vi "specu1a 1.0.0 PInfo String to PInfo Cluster.vi"(1 "Unit Information in":T1) -> (0 "output cluster":T2)   [LabVIEW 2010]
uses:
  Controls/specu1a 1.0.0 Product Information.ctl
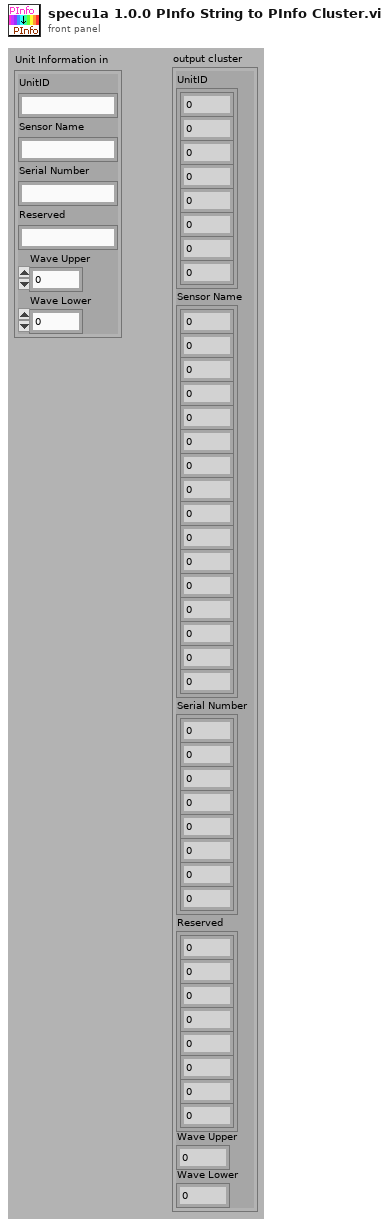
[diagram p1: front panel]
types:
  T1 = typedef "specu1a 1.0.0 Product Information.ctl" = cluster{"UnitID":string, "Sensor Name":string, "Serial Number":string, "Reserved":string, "Wave Upper":u16, "Wave Lower":u16}
  T2 = cluster{"UnitID":cluster{u8, u8, u8, u8, u8, u8, u8, u8}, "Sensor Name":cluster{u8, u8, u8, u8, u8, u8, u8, u8, u8, u8, u8, u8, u8, u8, u8, u8}, "Serial Number":cluster{u8, u8, u8, u8, u8, u8, u8, u8}, "Reserved":cluster{u8, u8, u8, u8, u8, u8, u8, u8}, "Wave Upper":u16, "Wave Lower":u16}
  T3 = cluster{u8, u8, u8, u8, u8, u8, u8, u8, u8, u8, u8, u8, u8, u8, u8, u8}
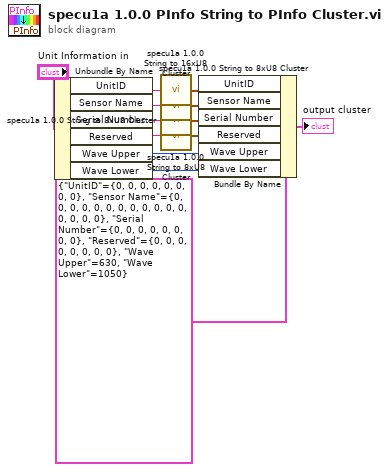
[diagram p0: block diagram]
diagram:
  n1 = Unbundle By Name("Unit Information in") -> ("UnitID"=w2:string, "Sensor Name"=w3:string, "Serial Number"=w4:string, "Reserved"=w5:string, "Wave Upper"=w10:u16, "Wave Lower"=w11:u16)
  n2 = call "specu1a 1.0.0 String to 8xU8 Cluster.vi"("String in"=w2) -> ("8xU8 Cluster"=w6:cluster{u8, u8, u8, u8, u8, u8, u8, u8})  [unwired: 14 in]
  n3 = call "specu1a 1.0.0 String to 16xU8 Cluster.vi"("String in"=w3) -> ("16xU8 Cluster"=w7:T3)  [unwired: 14 in]
  n4 = call "specu1a 1.0.0 String to 8xU8 Cluster.vi"("String in"=w4) -> ("8xU8 Cluster"=w9:cluster{u8, u8, u8, u8, u8, u8, u8, u8})  [unwired: 14 in]
  n5 = call "specu1a 1.0.0 String to 8xU8 Cluster.vi"("String in"=w5) -> ("8xU8 Cluster"=w8:cluster{u8, u8, u8, u8, u8, u8, u8, u8})  [unwired: 14 in]
  n6 = Bundle By Name(cluster=T2 {"UnitID"={0, 0, 0, 0, 0, 0, 0, 0}, "Sensor Name"={0, 0, 0, 0, 0, 0, 0, 0, 0, 0, 0, 0, 0, 0, 0, 0}, "Serial Number"={0, 0, 0, 0, 0, 0, 0, 0}, "Reserved"={0, 0, 0, 0, 0, 0, 0, 0}, "Wave Upper"=630, "Wave Lower"=1050} ("output cluster"), "UnitID"=w6, "Sensor Name"=w7, "Serial Number"=w9, "Reserved"=w8, "Wave Upper"=w10, "Wave Lower"=w11) -> (→"output cluster":T2)
